vi "Edit_Maths_Equation.vi"(3 "Template Info Array":T1[](array[typedef]) {"Tolerance" min=0.0 format="%#.4f"}, 4 "Maths Equation In":string, 5 "Channel Name":string) -> (0 "Template Info Array Out":T1[](array[typedef]) {"Tolerance" min=0.0 format="%#.4f"}, 1 "Maths Equation Out":string)   [LabVIEW 2013]
uses:
  File_Template_Clus.ctl
panel:
  out "Maths Equation Symbols":string
  in  "Start String":string
  in  "K":u16(ring) items=["Survey:No:", "U(ref)::", "U(ref):Turb:%", "U_{5hp}/U_{ref}::", "Vmag_{5hp}::", "U_{5hp}::", "V_{5hp}::", "W_{5hp}::", "Y_{5hp} (mm)::", "Z_{5hp} (mm)::", "U_{HW}::", "U_{HW}/U_{ref}::", "U_{HW}:Turb:%", "Y_{HW} (mm)::", "Z_{HW} (mm)::", "Date:of:Measurement", "Time:Measurement:Commenced", "Run:Start Time:", "Seconds:since:1st Jan", "Run:Messages:", "Original:Results:Filename", "Raw:Data:Filename", "Reference:Temperature:Used for Corrections", "Atmos:Pressure:Used for Corrections", "Slab Metadata:X-Location:", "Slab Metadata:Floor:", "Slab Metadata:Diverters:", "Slab Metadata:Screens:", "Slab Metadata:TurningVanes:", "Slab Metadata:Deflectors:", "Slab Metadata:MirrorWall:", "Slab Metadata:CloudWall:", "Slab Metadata:DiffuserExit:", "Slab Metadata:ConfigNumber:", "Slab Metadata:ProfileXLocation:", "Slab Metadata:DivererAngle:", "Slab Metadata:DiverterOrientation:", "Slab Metadata:DiverterAngleUpper:", "Slab Metadata:DiverterAngleLower:", "Slab Metadata:DiverterOrientUpper:", "Slab Metadata:DiverterOrientLower:", "Slab Metadata:MirrorWallStandoff:", "Slab Metadata:VertDivWall:", "Slab Metadata:VertDivWindow:", "Ch 0:Variance:Gen (Uref)", "Ch 6:Variance:HW (HW)", "Gen (Uref):Standard Error:in Mean", "Gen (Uref):Standard Error:in Variance", "Ch 1:Mean:Mano (5-1)", "Ch 1:Variance:Mano (5-1)", "Ch 1:SD:Mano (5-1)", "Ch 1:SDonMean:Mano (5-1)", "Ch 2:Mean:Mano (5-2)", "Ch 2:Variance:Mano (5-2)", "Ch 3:Mean:Mano (5-3)", "Ch 3:Variance:Mano (5-3)", "Ch 4:Mean:Mano (5-4)", "Ch 4:Variance:Mano (5-4)", "Ch 5:Mean:Mano (5-5)", "Ch 5:Variance:Mano (5-5)", "HW (HW):Standard Error:in Mean", "HW (HW):Standard Error:in Variance", "HW (HW):Timescale Estimate:Integrated to 25%", "Mode:Plug in:"]
  in  "String 10":string
  in  "J":u16(ring) items=["Survey:No:", "U(ref)::", "U(ref):Turb:%", "U_{5hp}/U_{ref}::", "Vmag_{5hp}::", "U_{5hp}::", "V_{5hp}::", "W_{5hp}::", "Y_{5hp} (mm)::", "Z_{5hp} (mm)::", "U_{HW}::", "U_{HW}/U_{ref}::", "U_{HW}:Turb:%", "Y_{HW} (mm)::", "Z_{HW} (mm)::", "Date:of:Measurement", "Time:Measurement:Commenced", "Run:Start Time:", "Seconds:since:1st Jan", "Run:Messages:", "Original:Results:Filename", "Raw:Data:Filename", "Reference:Temperature:Used for Corrections", "Atmos:Pressure:Used for Corrections", "Slab Metadata:X-Location:", "Slab Metadata:Floor:", "Slab Metadata:Diverters:", "Slab Metadata:Screens:", "Slab Metadata:TurningVanes:", "Slab Metadata:Deflectors:", "Slab Metadata:MirrorWall:", "Slab Metadata:CloudWall:", "Slab Metadata:DiffuserExit:", "Slab Metadata:ConfigNumber:", "Slab Metadata:ProfileXLocation:", "Slab Metadata:DivererAngle:", "Slab Metadata:DiverterOrientation:", "Slab Metadata:DiverterAngleUpper:", "Slab Metadata:DiverterAngleLower:", "Slab Metadata:DiverterOrientUpper:", "Slab Metadata:DiverterOrientLower:", "Slab Metadata:MirrorWallStandoff:", "Slab Metadata:VertDivWall:", "Slab Metadata:VertDivWindow:", "Ch 0:Variance:Gen (Uref)", "Ch 6:Variance:HW (HW)", "Gen (Uref):Standard Error:in Mean", "Gen (Uref):Standard Error:in Variance", "Ch 1:Mean:Mano (5-1)", "Ch 1:Variance:Mano (5-1)", "Ch 1:SD:Mano (5-1)", "Ch 1:SDonMean:Mano (5-1)", "Ch 2:Mean:Mano (5-2)", "Ch 2:Variance:Mano (5-2)", "Ch 3:Mean:Mano (5-3)", "Ch 3:Variance:Mano (5-3)", "Ch 4:Mean:Mano (5-4)", "Ch 4:Variance:Mano (5-4)", "Ch 5:Mean:Mano (5-5)", "Ch 5:Variance:Mano (5-5)", "HW (HW):Standard Error:in Mean", "HW (HW):Standard Error:in Variance", "HW (HW):Timescale Estimate:Integrated to 25%", "Mode:Plug in:"]
  in  "String 9":string
  in  "H":u16(ring) items=["Survey:No:", "U(ref)::", "U(ref):Turb:%", "U_{5hp}/U_{ref}::", "Vmag_{5hp}::", "U_{5hp}::", "V_{5hp}::", "W_{5hp}::", "Y_{5hp} (mm)::", "Z_{5hp} (mm)::", "U_{HW}::", "U_{HW}/U_{ref}::", "U_{HW}:Turb:%", "Y_{HW} (mm)::", "Z_{HW} (mm)::", "Date:of:Measurement", "Time:Measurement:Commenced", "Run:Start Time:", "Seconds:since:1st Jan", "Run:Messages:", "Original:Results:Filename", "Raw:Data:Filename", "Reference:Temperature:Used for Corrections", "Atmos:Pressure:Used for Corrections", "Slab Metadata:X-Location:", "Slab Metadata:Floor:", "Slab Metadata:Diverters:", "Slab Metadata:Screens:", "Slab Metadata:TurningVanes:", "Slab Metadata:Deflectors:", "Slab Metadata:MirrorWall:", "Slab Metadata:CloudWall:", "Slab Metadata:DiffuserExit:", "Slab Metadata:ConfigNumber:", "Slab Metadata:ProfileXLocation:", "Slab Metadata:DivererAngle:", "Slab Metadata:DiverterOrientation:", "Slab Metadata:DiverterAngleUpper:", "Slab Metadata:DiverterAngleLower:", "Slab Metadata:DiverterOrientUpper:", "Slab Metadata:DiverterOrientLower:", "Slab Metadata:MirrorWallStandoff:", "Slab Metadata:VertDivWall:", "Slab Metadata:VertDivWindow:", "Ch 0:Variance:Gen (Uref)", "Ch 6:Variance:HW (HW)", "Gen (Uref):Standard Error:in Mean", "Gen (Uref):Standard Error:in Variance", "Ch 1:Mean:Mano (5-1)", "Ch 1:Variance:Mano (5-1)", "Ch 1:SD:Mano (5-1)", "Ch 1:SDonMean:Mano (5-1)", "Ch 2:Mean:Mano (5-2)", "Ch 2:Variance:Mano (5-2)", "Ch 3:Mean:Mano (5-3)", "Ch 3:Variance:Mano (5-3)", "Ch 4:Mean:Mano (5-4)", "Ch 4:Variance:Mano (5-4)", "Ch 5:Mean:Mano (5-5)", "Ch 5:Variance:Mano (5-5)", "HW (HW):Standard Error:in Mean", "HW (HW):Standard Error:in Variance", "HW (HW):Timescale Estimate:Integrated to 25%", "Mode:Plug in:"]
  in  "String 8":string
  in  "G":u16(ring) items=["Survey:No:", "U(ref)::", "U(ref):Turb:%", "U_{5hp}/U_{ref}::", "Vmag_{5hp}::", "U_{5hp}::", "V_{5hp}::", "W_{5hp}::", "Y_{5hp} (mm)::", "Z_{5hp} (mm)::", "U_{HW}::", "U_{HW}/U_{ref}::", "U_{HW}:Turb:%", "Y_{HW} (mm)::", "Z_{HW} (mm)::", "Date:of:Measurement", "Time:Measurement:Commenced", "Run:Start Time:", "Seconds:since:1st Jan", "Run:Messages:", "Original:Results:Filename", "Raw:Data:Filename", "Reference:Temperature:Used for Corrections", "Atmos:Pressure:Used for Corrections", "Slab Metadata:X-Location:", "Slab Metadata:Floor:", "Slab Metadata:Diverters:", "Slab Metadata:Screens:", "Slab Metadata:TurningVanes:", "Slab Metadata:Deflectors:", "Slab Metadata:MirrorWall:", "Slab Metadata:CloudWall:", "Slab Metadata:DiffuserExit:", "Slab Metadata:ConfigNumber:", "Slab Metadata:ProfileXLocation:", "Slab Metadata:DivererAngle:", "Slab Metadata:DiverterOrientation:", "Slab Metadata:DiverterAngleUpper:", "Slab Metadata:DiverterAngleLower:", "Slab Metadata:DiverterOrientUpper:", "Slab Metadata:DiverterOrientLower:", "Slab Metadata:MirrorWallStandoff:", "Slab Metadata:VertDivWall:", "Slab Metadata:VertDivWindow:", "Ch 0:Variance:Gen (Uref)", "Ch 6:Variance:HW (HW)", "Gen (Uref):Standard Error:in Mean", "Gen (Uref):Standard Error:in Variance", "Ch 1:Mean:Mano (5-1)", "Ch 1:Variance:Mano (5-1)", "Ch 1:SD:Mano (5-1)", "Ch 1:SDonMean:Mano (5-1)", "Ch 2:Mean:Mano (5-2)", "Ch 2:Variance:Mano (5-2)", "Ch 3:Mean:Mano (5-3)", "Ch 3:Variance:Mano (5-3)", "Ch 4:Mean:Mano (5-4)", "Ch 4:Variance:Mano (5-4)", "Ch 5:Mean:Mano (5-5)", "Ch 5:Variance:Mano (5-5)", "HW (HW):Standard Error:in Mean", "HW (HW):Standard Error:in Variance", "HW (HW):Timescale Estimate:Integrated to 25%", "Mode:Plug in:"]
  in  "String 7":string
  in  "F":u16(ring) items=["Survey:No:", "U(ref)::", "U(ref):Turb:%", "U_{5hp}/U_{ref}::", "Vmag_{5hp}::", "U_{5hp}::", "V_{5hp}::", "W_{5hp}::", "Y_{5hp} (mm)::", "Z_{5hp} (mm)::", "U_{HW}::", "U_{HW}/U_{ref}::", "U_{HW}:Turb:%", "Y_{HW} (mm)::", "Z_{HW} (mm)::", "Date:of:Measurement", "Time:Measurement:Commenced", "Run:Start Time:", "Seconds:since:1st Jan", "Run:Messages:", "Original:Results:Filename", "Raw:Data:Filename", "Reference:Temperature:Used for Corrections", "Atmos:Pressure:Used for Corrections", "Slab Metadata:X-Location:", "Slab Metadata:Floor:", "Slab Metadata:Diverters:", "Slab Metadata:Screens:", "Slab Metadata:TurningVanes:", "Slab Metadata:Deflectors:", "Slab Metadata:MirrorWall:", "Slab Metadata:CloudWall:", "Slab Metadata:DiffuserExit:", "Slab Metadata:ConfigNumber:", "Slab Metadata:ProfileXLocation:", "Slab Metadata:DivererAngle:", "Slab Metadata:DiverterOrientation:", "Slab Metadata:DiverterAngleUpper:", "Slab Metadata:DiverterAngleLower:", "Slab Metadata:DiverterOrientUpper:", "Slab Metadata:DiverterOrientLower:", "Slab Metadata:MirrorWallStandoff:", "Slab Metadata:VertDivWall:", "Slab Metadata:VertDivWindow:", "Ch 0:Variance:Gen (Uref)", "Ch 6:Variance:HW (HW)", "Gen (Uref):Standard Error:in Mean", "Gen (Uref):Standard Error:in Variance", "Ch 1:Mean:Mano (5-1)", "Ch 1:Variance:Mano (5-1)", "Ch 1:SD:Mano (5-1)", "Ch 1:SDonMean:Mano (5-1)", "Ch 2:Mean:Mano (5-2)", "Ch 2:Variance:Mano (5-2)", "Ch 3:Mean:Mano (5-3)", "Ch 3:Variance:Mano (5-3)", "Ch 4:Mean:Mano (5-4)", "Ch 4:Variance:Mano (5-4)", "Ch 5:Mean:Mano (5-5)", "Ch 5:Variance:Mano (5-5)", "HW (HW):Standard Error:in Mean", "HW (HW):Standard Error:in Variance", "HW (HW):Timescale Estimate:Integrated to 25%", "Mode:Plug in:"]
  in  "String 6":string
  in  "E":u16(ring) items=["Survey:No:", "U(ref)::", "U(ref):Turb:%", "U_{5hp}/U_{ref}::", "Vmag_{5hp}::", "U_{5hp}::", "V_{5hp}::", "W_{5hp}::", "Y_{5hp} (mm)::", "Z_{5hp} (mm)::", "U_{HW}::", "U_{HW}/U_{ref}::", "U_{HW}:Turb:%", "Y_{HW} (mm)::", "Z_{HW} (mm)::", "Date:of:Measurement", "Time:Measurement:Commenced", "Run:Start Time:", "Seconds:since:1st Jan", "Run:Messages:", "Original:Results:Filename", "Raw:Data:Filename", "Reference:Temperature:Used for Corrections", "Atmos:Pressure:Used for Corrections", "Slab Metadata:X-Location:", "Slab Metadata:Floor:", "Slab Metadata:Diverters:", "Slab Metadata:Screens:", "Slab Metadata:TurningVanes:", "Slab Metadata:Deflectors:", "Slab Metadata:MirrorWall:", "Slab Metadata:CloudWall:", "Slab Metadata:DiffuserExit:", "Slab Metadata:ConfigNumber:", "Slab Metadata:ProfileXLocation:", "Slab Metadata:DivererAngle:", "Slab Metadata:DiverterOrientation:", "Slab Metadata:DiverterAngleUpper:", "Slab Metadata:DiverterAngleLower:", "Slab Metadata:DiverterOrientUpper:", "Slab Metadata:DiverterOrientLower:", "Slab Metadata:MirrorWallStandoff:", "Slab Metadata:VertDivWall:", "Slab Metadata:VertDivWindow:", "Ch 0:Variance:Gen (Uref)", "Ch 6:Variance:HW (HW)", "Gen (Uref):Standard Error:in Mean", "Gen (Uref):Standard Error:in Variance", "Ch 1:Mean:Mano (5-1)", "Ch 1:Variance:Mano (5-1)", "Ch 1:SD:Mano (5-1)", "Ch 1:SDonMean:Mano (5-1)", "Ch 2:Mean:Mano (5-2)", "Ch 2:Variance:Mano (5-2)", "Ch 3:Mean:Mano (5-3)", "Ch 3:Variance:Mano (5-3)", "Ch 4:Mean:Mano (5-4)", "Ch 4:Variance:Mano (5-4)", "Ch 5:Mean:Mano (5-5)", "Ch 5:Variance:Mano (5-5)", "HW (HW):Standard Error:in Mean", "HW (HW):Standard Error:in Variance", "HW (HW):Timescale Estimate:Integrated to 25%", "Mode:Plug in:"]
  in  "String 5":string
  in  "D":u16(ring) items=["Survey:No:", "U(ref)::", "U(ref):Turb:%", "U_{5hp}/U_{ref}::", "Vmag_{5hp}::", "U_{5hp}::", "V_{5hp}::", "W_{5hp}::", "Y_{5hp} (mm)::", "Z_{5hp} (mm)::", "U_{HW}::", "U_{HW}/U_{ref}::", "U_{HW}:Turb:%", "Y_{HW} (mm)::", "Z_{HW} (mm)::", "Date:of:Measurement", "Time:Measurement:Commenced", "Run:Start Time:", "Seconds:since:1st Jan", "Run:Messages:", "Original:Results:Filename", "Raw:Data:Filename", "Reference:Temperature:Used for Corrections", "Atmos:Pressure:Used for Corrections", "Slab Metadata:X-Location:", "Slab Metadata:Floor:", "Slab Metadata:Diverters:", "Slab Metadata:Screens:", "Slab Metadata:TurningVanes:", "Slab Metadata:Deflectors:", "Slab Metadata:MirrorWall:", "Slab Metadata:CloudWall:", "Slab Metadata:DiffuserExit:", "Slab Metadata:ConfigNumber:", "Slab Metadata:ProfileXLocation:", "Slab Metadata:DivererAngle:", "Slab Metadata:DiverterOrientation:", "Slab Metadata:DiverterAngleUpper:", "Slab Metadata:DiverterAngleLower:", "Slab Metadata:DiverterOrientUpper:", "Slab Metadata:DiverterOrientLower:", "Slab Metadata:MirrorWallStandoff:", "Slab Metadata:VertDivWall:", "Slab Metadata:VertDivWindow:", "Ch 0:Variance:Gen (Uref)", "Ch 6:Variance:HW (HW)", "Gen (Uref):Standard Error:in Mean", "Gen (Uref):Standard Error:in Variance", "Ch 1:Mean:Mano (5-1)", "Ch 1:Variance:Mano (5-1)", "Ch 1:SD:Mano (5-1)", "Ch 1:SDonMean:Mano (5-1)", "Ch 2:Mean:Mano (5-2)", "Ch 2:Variance:Mano (5-2)", "Ch 3:Mean:Mano (5-3)", "Ch 3:Variance:Mano (5-3)", "Ch 4:Mean:Mano (5-4)", "Ch 4:Variance:Mano (5-4)", "Ch 5:Mean:Mano (5-5)", "Ch 5:Variance:Mano (5-5)", "HW (HW):Standard Error:in Mean", "HW (HW):Standard Error:in Variance", "HW (HW):Timescale Estimate:Integrated to 25%", "Mode:Plug in:"]
  in  "String 4":string
  in  "C":u16(ring) items=["Survey:No:", "U(ref)::", "U(ref):Turb:%", "U_{5hp}/U_{ref}::", "Vmag_{5hp}::", "U_{5hp}::", "V_{5hp}::", "W_{5hp}::", "Y_{5hp} (mm)::", "Z_{5hp} (mm)::", "U_{HW}::", "U_{HW}/U_{ref}::", "U_{HW}:Turb:%", "Y_{HW} (mm)::", "Z_{HW} (mm)::", "Date:of:Measurement", "Time:Measurement:Commenced", "Run:Start Time:", "Seconds:since:1st Jan", "Run:Messages:", "Original:Results:Filename", "Raw:Data:Filename", "Reference:Temperature:Used for Corrections", "Atmos:Pressure:Used for Corrections", "Slab Metadata:X-Location:", "Slab Metadata:Floor:", "Slab Metadata:Diverters:", "Slab Metadata:Screens:", "Slab Metadata:TurningVanes:", "Slab Metadata:Deflectors:", "Slab Metadata:MirrorWall:", "Slab Metadata:CloudWall:", "Slab Metadata:DiffuserExit:", "Slab Metadata:ConfigNumber:", "Slab Metadata:ProfileXLocation:", "Slab Metadata:DivererAngle:", "Slab Metadata:DiverterOrientation:", "Slab Metadata:DiverterAngleUpper:", "Slab Metadata:DiverterAngleLower:", "Slab Metadata:DiverterOrientUpper:", "Slab Metadata:DiverterOrientLower:", "Slab Metadata:MirrorWallStandoff:", "Slab Metadata:VertDivWall:", "Slab Metadata:VertDivWindow:", "Ch 0:Variance:Gen (Uref)", "Ch 6:Variance:HW (HW)", "Gen (Uref):Standard Error:in Mean", "Gen (Uref):Standard Error:in Variance", "Ch 1:Mean:Mano (5-1)", "Ch 1:Variance:Mano (5-1)", "Ch 1:SD:Mano (5-1)", "Ch 1:SDonMean:Mano (5-1)", "Ch 2:Mean:Mano (5-2)", "Ch 2:Variance:Mano (5-2)", "Ch 3:Mean:Mano (5-3)", "Ch 3:Variance:Mano (5-3)", "Ch 4:Mean:Mano (5-4)", "Ch 4:Variance:Mano (5-4)", "Ch 5:Mean:Mano (5-5)", "Ch 5:Variance:Mano (5-5)", "HW (HW):Standard Error:in Mean", "HW (HW):Standard Error:in Variance", "HW (HW):Timescale Estimate:Integrated to 25%", "Mode:Plug in:"]
  in  "String 3":string
  in  "B":u16(ring) items=["Survey:No:", "U(ref)::", "U(ref):Turb:%", "U_{5hp}/U_{ref}::", "Vmag_{5hp}::", "U_{5hp}::", "V_{5hp}::", "W_{5hp}::", "Y_{5hp} (mm)::", "Z_{5hp} (mm)::", "U_{HW}::", "U_{HW}/U_{ref}::", "U_{HW}:Turb:%", "Y_{HW} (mm)::", "Z_{HW} (mm)::", "Date:of:Measurement", "Time:Measurement:Commenced", "Run:Start Time:", "Seconds:since:1st Jan", "Run:Messages:", "Original:Results:Filename", "Raw:Data:Filename", "Reference:Temperature:Used for Corrections", "Atmos:Pressure:Used for Corrections", "Slab Metadata:X-Location:", "Slab Metadata:Floor:", "Slab Metadata:Diverters:", "Slab Metadata:Screens:", "Slab Metadata:TurningVanes:", "Slab Metadata:Deflectors:", "Slab Metadata:MirrorWall:", "Slab Metadata:CloudWall:", "Slab Metadata:DiffuserExit:", "Slab Metadata:ConfigNumber:", "Slab Metadata:ProfileXLocation:", "Slab Metadata:DivererAngle:", "Slab Metadata:DiverterOrientation:", "Slab Metadata:DiverterAngleUpper:", "Slab Metadata:DiverterAngleLower:", "Slab Metadata:DiverterOrientUpper:", "Slab Metadata:DiverterOrientLower:", "Slab Metadata:MirrorWallStandoff:", "Slab Metadata:VertDivWall:", "Slab Metadata:VertDivWindow:", "Ch 0:Variance:Gen (Uref)", "Ch 6:Variance:HW (HW)", "Gen (Uref):Standard Error:in Mean", "Gen (Uref):Standard Error:in Variance", "Ch 1:Mean:Mano (5-1)", "Ch 1:Variance:Mano (5-1)", "Ch 1:SD:Mano (5-1)", "Ch 1:SDonMean:Mano (5-1)", "Ch 2:Mean:Mano (5-2)", "Ch 2:Variance:Mano (5-2)", "Ch 3:Mean:Mano (5-3)", "Ch 3:Variance:Mano (5-3)", "Ch 4:Mean:Mano (5-4)", "Ch 4:Variance:Mano (5-4)", "Ch 5:Mean:Mano (5-5)", "Ch 5:Variance:Mano (5-5)", "HW (HW):Standard Error:in Mean", "HW (HW):Standard Error:in Variance", "HW (HW):Timescale Estimate:Integrated to 25%", "Mode:Plug in:"]
  in  "String 2":string
  in  "A":u16(ring) items=["Survey:No:", "U(ref)::", "U(ref):Turb:%", "U_{5hp}/U_{ref}::", "Vmag_{5hp}::", "U_{5hp}::", "V_{5hp}::", "W_{5hp}::", "Y_{5hp} (mm)::", "Z_{5hp} (mm)::", "U_{HW}::", "U_{HW}/U_{ref}::", "U_{HW}:Turb:%", "Y_{HW} (mm)::", "Z_{HW} (mm)::", "Date:of:Measurement", "Time:Measurement:Commenced", "Run:Start Time:", "Seconds:since:1st Jan", "Run:Messages:", "Original:Results:Filename", "Raw:Data:Filename", "Reference:Temperature:Used for Corrections", "Atmos:Pressure:Used for Corrections", "Slab Metadata:X-Location:", "Slab Metadata:Floor:", "Slab Metadata:Diverters:", "Slab Metadata:Screens:", "Slab Metadata:TurningVanes:", "Slab Metadata:Deflectors:", "Slab Metadata:MirrorWall:", "Slab Metadata:CloudWall:", "Slab Metadata:DiffuserExit:", "Slab Metadata:ConfigNumber:", "Slab Metadata:ProfileXLocation:", "Slab Metadata:DivererAngle:", "Slab Metadata:DiverterOrientation:", "Slab Metadata:DiverterAngleUpper:", "Slab Metadata:DiverterAngleLower:", "Slab Metadata:DiverterOrientUpper:", "Slab Metadata:DiverterOrientLower:", "Slab Metadata:MirrorWallStandoff:", "Slab Metadata:VertDivWall:", "Slab Metadata:VertDivWindow:", "Ch 0:Variance:Gen (Uref)", "Ch 6:Variance:HW (HW)", "Gen (Uref):Standard Error:in Mean", "Gen (Uref):Standard Error:in Variance", "Ch 1:Mean:Mano (5-1)", "Ch 1:Variance:Mano (5-1)", "Ch 1:SD:Mano (5-1)", "Ch 1:SDonMean:Mano (5-1)", "Ch 2:Mean:Mano (5-2)", "Ch 2:Variance:Mano (5-2)", "Ch 3:Mean:Mano (5-3)", "Ch 3:Variance:Mano (5-3)", "Ch 4:Mean:Mano (5-4)", "Ch 4:Variance:Mano (5-4)", "Ch 5:Mean:Mano (5-5)", "Ch 5:Variance:Mano (5-5)", "HW (HW):Standard Error:in Mean", "HW (HW):Standard Error:in Variance", "HW (HW):Timescale Estimate:Integrated to 25%", "Mode:Plug in:"]
  in  "String 1":string
  in  "Reset":bool
  in  "Number of Variables":i32
  in  "OK":bool
  # "> 20  or\n<20   or\n =20"
  # "<<Characters_to_Match>>  <<Replace_Whole_String_with_this>>"
  # "<<Channel_Name>> contains <<Characters to match>> or\n<<Channel_Name>> does not contain <<Characters to match>>"
  # "<<Channel_Name_A>> + <<Channel_Name_B>> or\nConcatenate <<Channel_Name_A>> and <<Channel_Name_B>>"
  # "> 20  or\n<20   or\n =20"
  # "<<Characters_to_Match>>  <<Replace_Whole_String_with_this>>"
  # "<<Channel_Name>> contains <<Characters to match>> or\n<<Channel_Name>> does not contain <<Characters to match>>"
  # "<<Channel_Name_A>> + <<Channel_Name_B>> or\nConcatenate <<Channel_Name_A>> and <<Channel_Name_B>>"
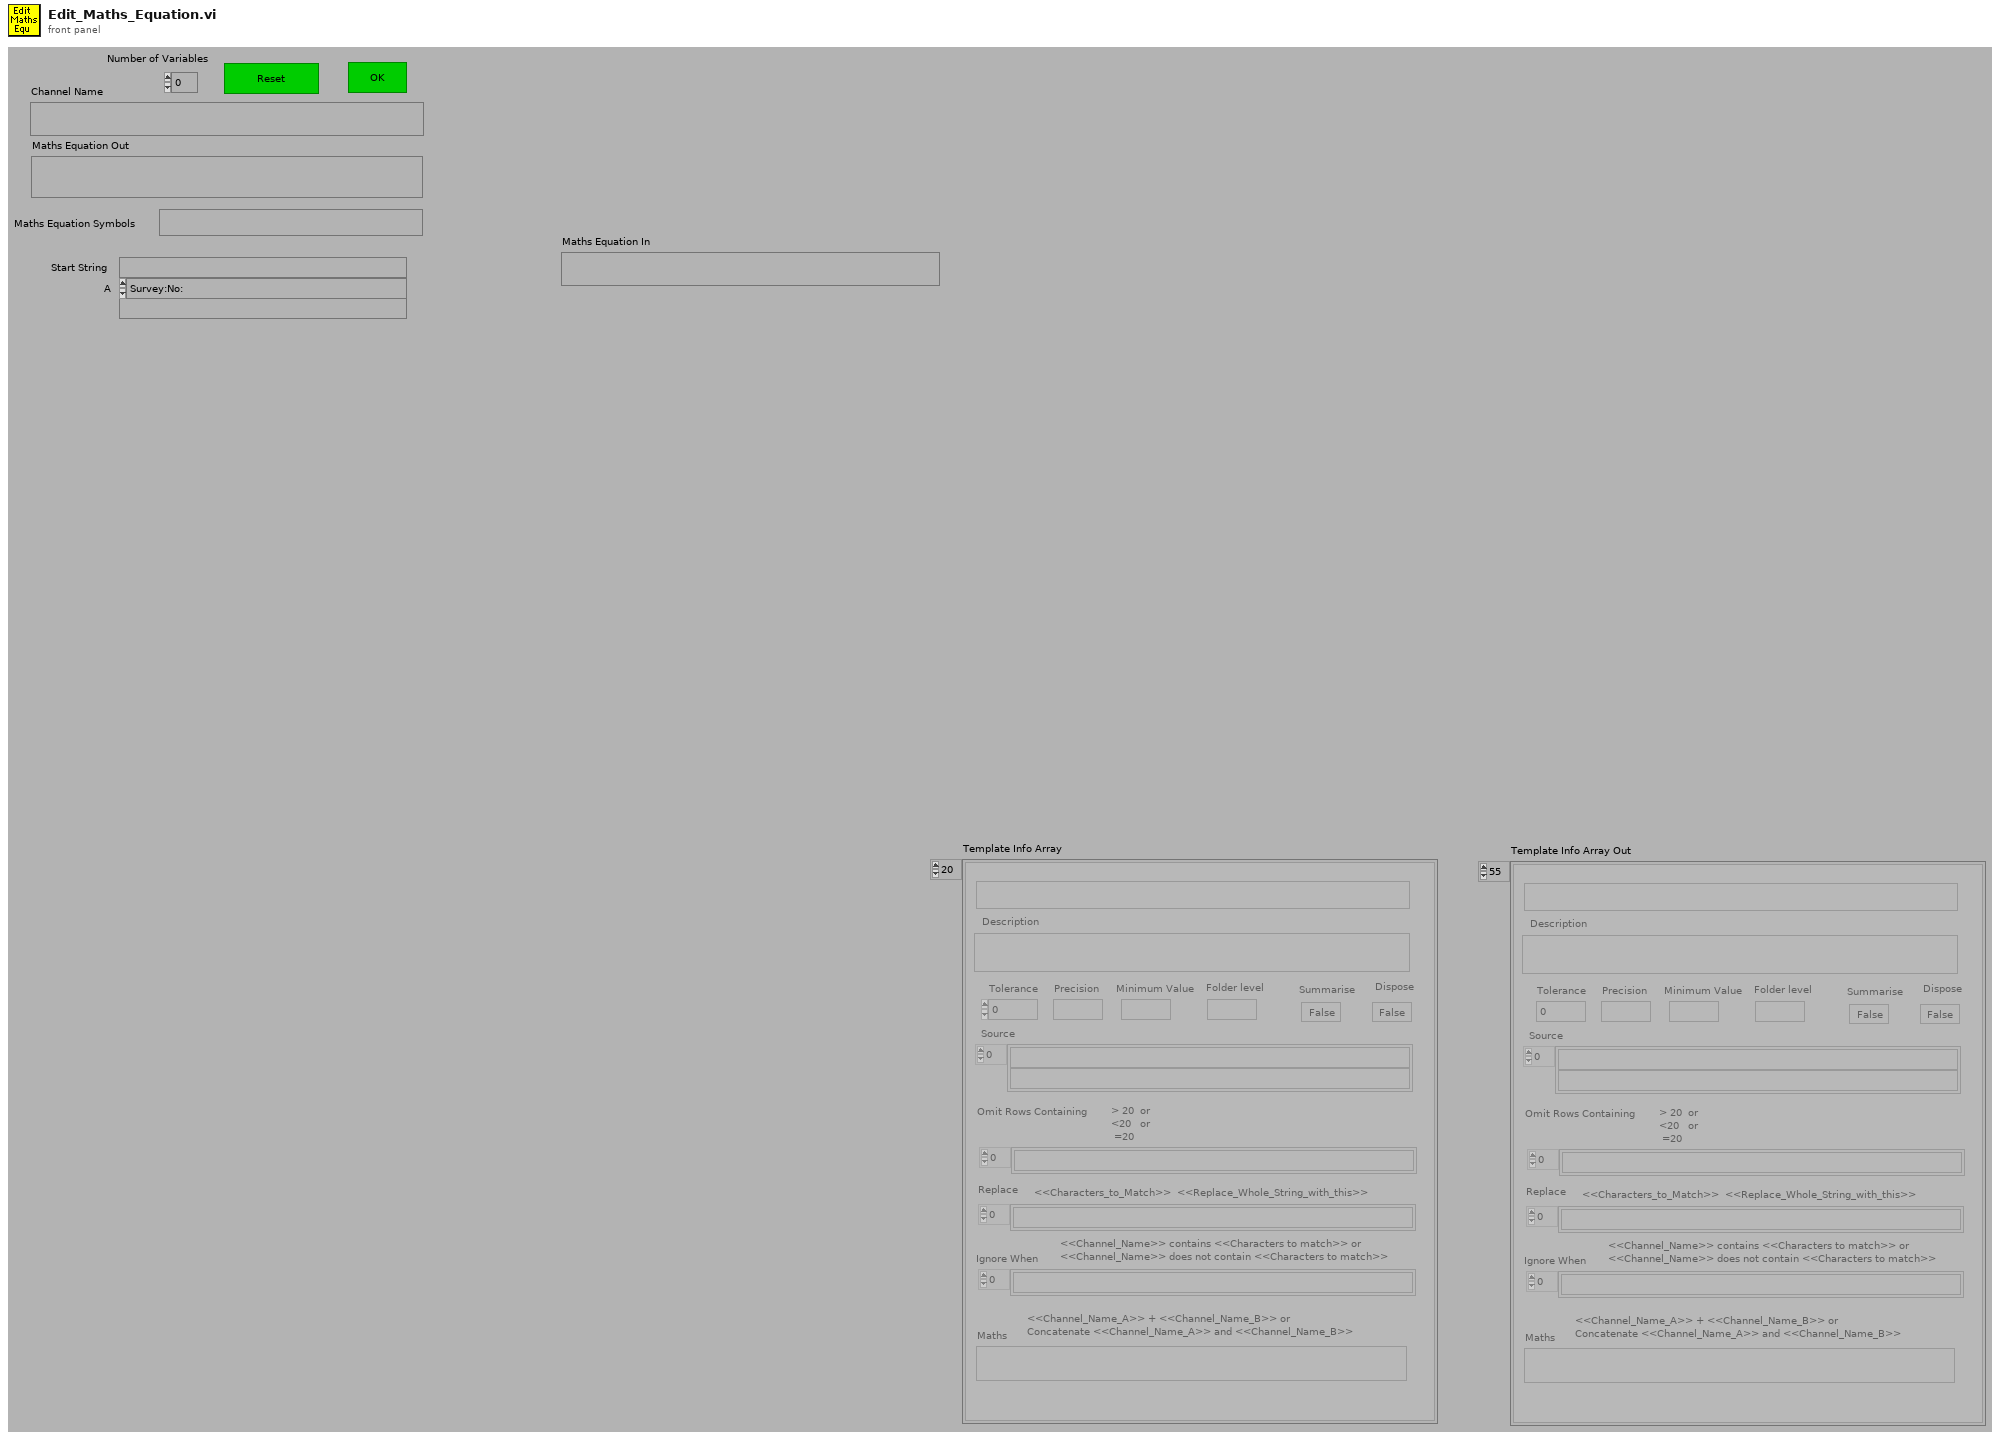
[diagram p1: front panel]
types:
  T1 = typedef "File_Template_Clus.ctl" = cluster{"Template Channel Name":string, "Description":string, "Tolerance":dbl, "Precision":string, "Folder level":string, "Source":string[], "Replace":string[], "Summarise":bool, "Dispose":bool, "Minimum Value":string, "Maths":string, "Omit Rows Containing":string[], "Ignore When":string[]}
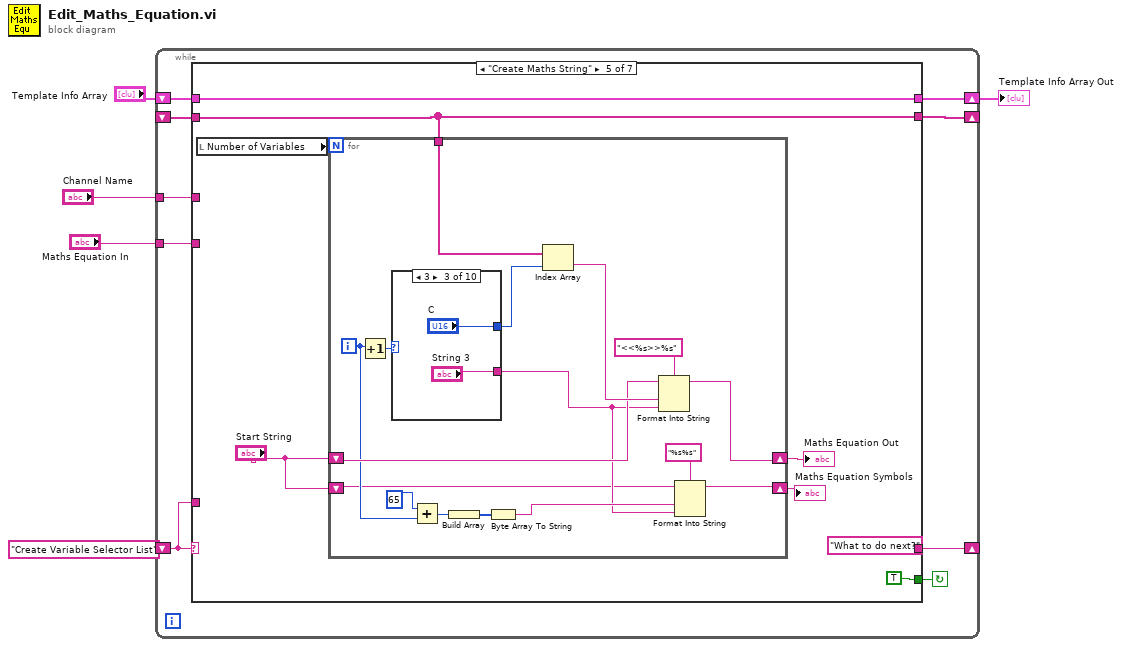
[diagram p0: block diagram]
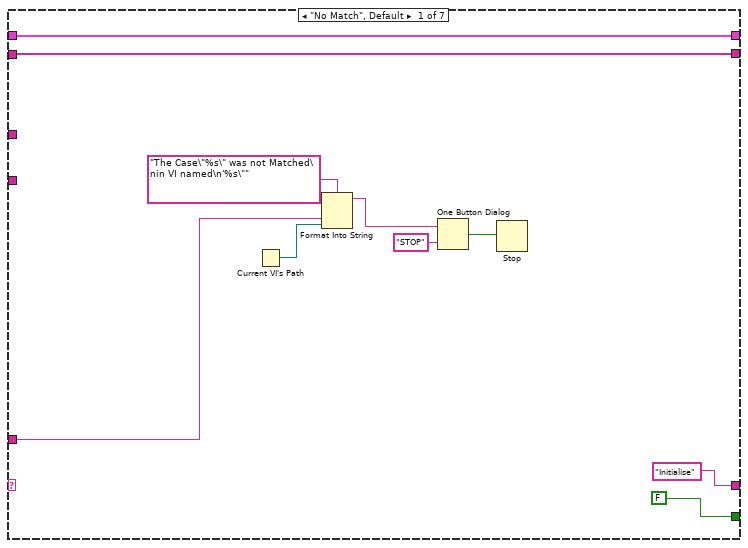
[diagram p2: hidden frame]
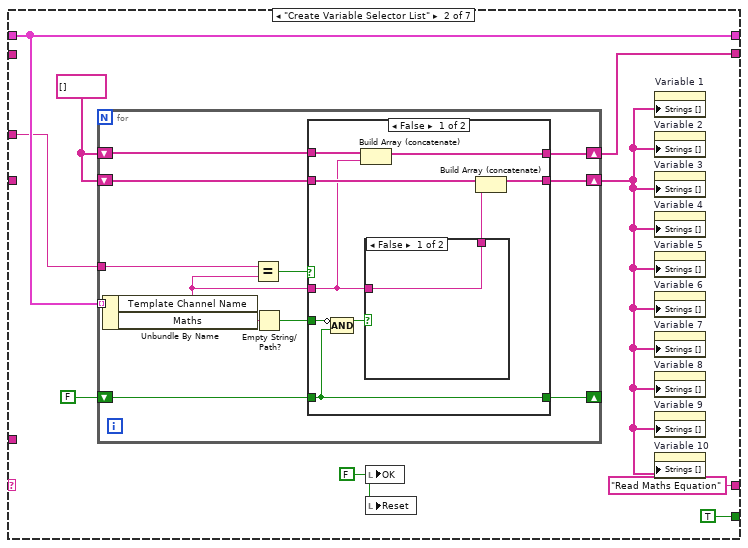
[diagram p3: hidden frame]
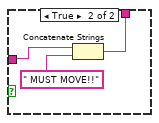
[diagram p4: hidden frame]
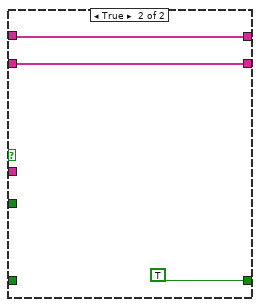
[diagram p5: hidden frame]
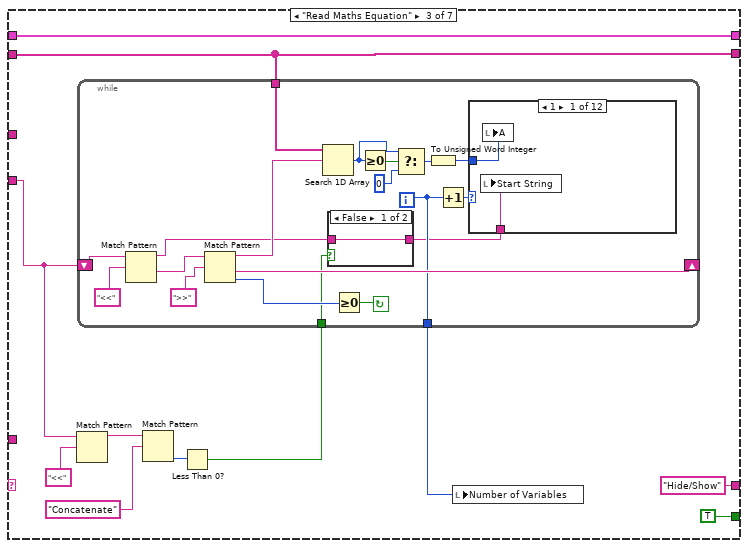
[diagram p6: hidden frame]
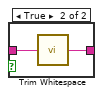
[diagram p7: hidden frame]
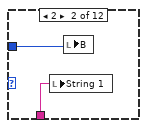
[diagram p8: hidden frame]
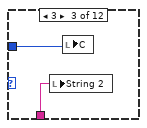
[diagram p9: hidden frame]
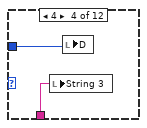
[diagram p10: hidden frame]
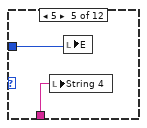
[diagram p11: hidden frame]
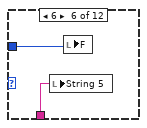
[diagram p12: hidden frame]
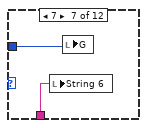
[diagram p13: hidden frame]
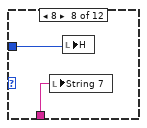
[diagram p14: hidden frame]
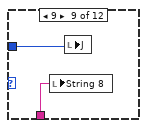
[diagram p15: hidden frame]
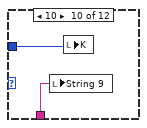
[diagram p16: hidden frame]
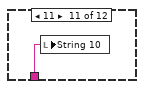
[diagram p17: hidden frame]
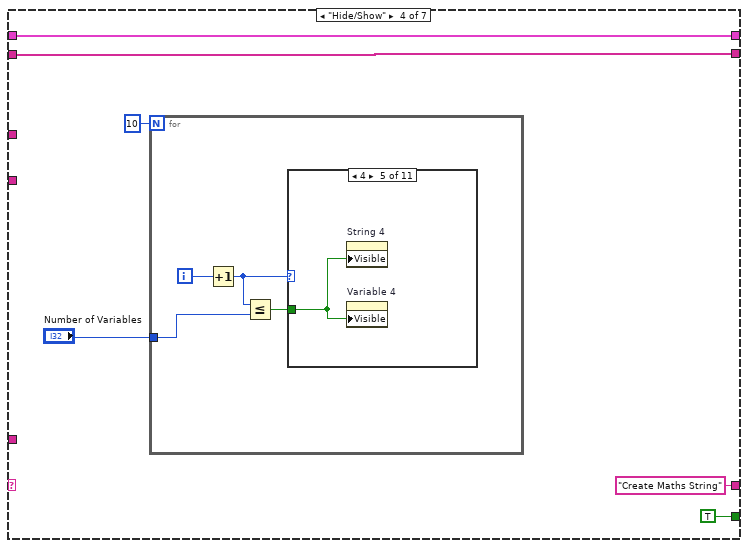
[diagram p19: hidden frame]
diagram:
  n1 = while {
    tunnel: "Channel Name" -> [w6]
    tunnel: "Maths Equation In" -> [w7]
    shift-left: _ -> [w8]
    shift-right: [w9] -> _
    shift-left: "Template Info Array" -> [w10]
    shift-right: [w11] -> w3
    shift-left: "Create Variable Selector List" -> [w12]
    shift-right: [w13] -> _
    stop <- w14 continue-if-true
    n2 = case shown="\"Create Maths String\"" w12 {
      tunnel: [FALSE TRUE TRUE TRUE TRUE TRUE FALSE] -> w14
      tunnel: ["Initialise" "Read Maths Equation" "Hide/Show" "Create Maths String" "What to do next?" w181 "End"] -> w13
      tunnel: w12 -> [w19 _ _ _ _ _ _]
      tunnel: [w16 w32 w71 w120 w141 w191 w200] -> w11
      tunnel: w10 -> [w16 w32 w71 w120 w141 w191 w200]
      tunnel: [w15 w30 w70 w119 w139 w185 w199] -> w9
      tunnel: w8 -> [w15 _ w70 w119 w139 w185 w199]
      tunnel: w7 -> [_ _ w66 _ _ _ _]
      tunnel: w6 -> [_ w31 _ _ _ _ _]
      frame "No Match", Default {
        n3 = Current VI's Path() -> (path=w18:path)
        n4 = Format Into String(format string="The Case\"%s\" was not Matched\nin VI named\n'%s\"" ("Format String"), w19, w18) -> (resulting string=w22:string)  [unwired: 2 in, 1 out]
        n5 = One Button Dialog(message=w22, button name ("OK")="STOP") -> (true=w20:bool)
        n6 = Stop(stop? (T)=w20) -> ()
      }
      frame "Create Variable Selector List" {
        w25 = FALSE ("OK")
        w28 = string[] []
        n7 = for {
          shift-right: [w40] -> w30
          shift-left: w28 -> [w42]
          shift-right: [w36] -> w27
          shift-left: w28 -> [w37]
          tunnel: w32 -> [w45] mode=indexing
          tunnel: w31 -> [w44]
          shift-right: [w35] -> _
          shift-left: FALSE -> [w34]
          n8 = Unbundle By Name(w45) -> ("Template Channel Name"=w41:string, "Maths"=w39:string)
          n9 = Equal?(x=w44, y=w41) -> (x = y?=w43:bool)
          n10 = Empty String/Path?(string/path=w39) -> (empty?=w38:bool)
          n11 = case shown="False" w43 {
            tunnel: w42 -> [w54 w60]
            tunnel: w41 -> [w49 _]
            tunnel: [w53 w60] -> w40
            tunnel: w38 -> [w48 _]
            tunnel: w37 -> [w52 w59]
            tunnel: [w51 w59] -> w36
            tunnel: [w46 TRUE] -> w35
            tunnel: w34 -> [w46 _]
            frame False {
              n12 = Compound Arithmetic op=AND(invert w48, w46) -> (w47:bool)
              n13 = Build Array (concatenate)(w54, w49) -> (w53:string[])
              n14 = case shown="False" w47 {
                tunnel: [w55 w57] -> w50
                tunnel: w49 -> [w55 w58]
                frame False {
                }
                frame True {
                  n15 = Concatenate Strings(w58, " MUST MOVE!!" ("Substring")) -> (w57:string)
                }
              }
              n16 = Build Array (concatenate)(w52, w50) -> (w51:string[])
            }
            frame True {
            }
          }
        }
        n17 = local write "OK"(w25) -> ()
        n18 = local write "Reset"(w25) -> ()
        n19 = property on="Variable 1" class="Ring (strict)"("Strings []"=w27) -> ()  [unwired: 2 in, 2 out]
        n20 = property on="Variable 2" class="Ring (strict)"("Strings []"=w27) -> ()  [unwired: 2 in, 2 out]
        n21 = property on="Variable 3" class="Ring (strict)"("Strings []"=w27) -> ()  [unwired: 2 in, 2 out]
        n22 = property on="Variable 4" class="Ring (strict)"("Strings []"=w27) -> ()  [unwired: 2 in, 2 out]
        n23 = property on="Variable 5" class="Ring (strict)"("Strings []"=w27) -> ()  [unwired: 2 in, 2 out]
        n24 = property on="Variable 6" class="Ring (strict)"("Strings []"=w27) -> ()  [unwired: 2 in, 2 out]
        n25 = property on="Variable 7" class="Ring (strict)"("Strings []"=w27) -> ()  [unwired: 2 in, 2 out]
        n26 = property on="Variable 8" class="Ring (strict)"("Strings []"=w27) -> ()  [unwired: 2 in, 2 out]
        n27 = property on="Variable 9" class="Ring (strict)"("Strings []"=w27) -> ()  [unwired: 2 in, 2 out]
        n28 = property on="Variable 10" class="Ring (strict)"("Strings []"=w27) -> ()  [unwired: 2 in, 2 out]
      }
      frame "Read Maths Equation" {
        n29 = Match Pattern(string=w66, regular expression="<<") -> (before substring=w65:string)  [unwired: 4 out]
        n30 = Match Pattern(string=w65, regular expression="Concatenate") -> (offset past match=w63:i32)  [unwired: 4 out]
        n31 = Less Than 0?(x=w63) -> (x < 0?=w62:bool)
        n32 = while {
          tunnel: [w79] -> w69
          tunnel: w70 -> [w88]
          shift-left: w66 -> [w91]
          shift-right: [w81] -> _
          tunnel: w62 -> [w73]
          i -> [w79]
          stop <- w89 continue-if-true
          n33 = Match Pattern(string=w91, regular expression="<<") -> (before substring=w77:string, after substring=w90:string)  [unwired: 3 out]
          n34 = Match Pattern(string=w90, regular expression=">>") -> (before substring=w87:string, after substring=w81:string, offset past match=w80:i32)  [unwired: 2 out]
          n35 = Search 1D Array(1D array=w88, element=w87) -> (index of element=w85:i32)  [unwired: 1 out]
          n36 = case shown="False" w73 {
            tunnel: w77 -> [w92 w94]
            tunnel: [w92 w93] -> w76
            frame False {
            }
            frame True {
              n37 = call <vilib>:"Trim Whitespace.vi"("string"=w94) -> ("trimmed string"=w93:string)  [unwired: 1 in]
            }
          }
          n38 = Greater Or Equal To 0?(x=w80) -> (x >= 0?=w89:bool)
          n39 = Greater Or Equal To 0?(x=w85) -> (x >= 0?=w86:bool)
          n40 = Select(t=w85, s=w86, f=0) -> (s? t:f=w82:i32)
          n41 = To Unsigned Word Integer(number=w82) -> (unsigned 16bit integer=w78:u16)
          n42 = Increment(x=w79) -> (x+1=w83:i32)
          n43 = case shown="1" w83 {
            tunnel: w78 -> [w96 w98 w100 w102 w104 w106 w108 w110 w112 w114 _ _]
            tunnel: w76 -> [w95 w97 w99 w101 w103 w105 w107 w109 w111 w113 w115 _]
            frame 1 {
              n44 = local write "Start String"(w95) -> ()
              n45 = local write "A"(w96) -> ()
            }
            frame 2 {
              n46 = local write "String 1"(w97) -> ()
              n47 = local write "B"(w98) -> ()
            }
            frame 3 {
              n48 = local write "String 2"(w99) -> ()
              n49 = local write "C"(w100) -> ()
            }
            frame 4 {
              n50 = local write "String 3"(w101) -> ()
              n51 = local write "D"(w102) -> ()
            }
            frame 5 {
              n52 = local write "String 4"(w103) -> ()
              n53 = local write "E"(w104) -> ()
            }
            frame 6 {
              n54 = local write "String 5"(w105) -> ()
              n55 = local write "F"(w106) -> ()
            }
            frame 7 {
              n56 = local write "String 6"(w107) -> ()
              n57 = local write "G"(w108) -> ()
            }
            frame 8 {
              n58 = local write "String 7"(w109) -> ()
              n59 = local write "H"(w110) -> ()
            }
            frame 9 {
              n60 = local write "String 8"(w111) -> ()
              n61 = local write "J"(w112) -> ()
            }
            frame 10 {
              n62 = local write "String 9"(w113) -> ()
              n63 = local write "K"(w114) -> ()
            }
            frame 11 {
              n64 = local write "String 10"(w115) -> ()
            }
            frame 12, Default {
            }
          }
        }
        n65 = local write "Number of Variables"(w69) -> ()
      }
      frame "Hide/Show" {
        n66 = for {
          N: 10 -> [_]
          tunnel: "Number of Variables" -> [w123]
          i -> [w125]
          n67 = Increment(x=w125) -> (x+1=w124:i32)
          n68 = Less Or Equal?(x=w124, y=w123) -> (x <= y?=w122:bool)
          n69 = case shown="4" w124 {
            tunnel: w122 -> [_ w126 w127 w128 w129 w130 w131 w132 w133 w134 w135]
            frame 0, Default {
            }
            frame 1 {
              n70 = property on="Variable 1" class="Ring (strict)"("Visible"=w126) -> ()  [unwired: 2 in, 2 out]
              n71 = property on="String 1" class="Str"("Visible"=w126) -> ()  [unwired: 2 in, 2 out]
            }
            frame 2 {
              n72 = property on="Variable 2" class="Ring (strict)"("Visible"=w127) -> ()  [unwired: 2 in, 2 out]
              n73 = property on="String 2" class="Str"("Visible"=w127) -> ()  [unwired: 2 in, 2 out]
            }
            frame 3 {
              n74 = property on="Variable 3" class="Ring (strict)"("Visible"=w128) -> ()  [unwired: 2 in, 2 out]
              n75 = property on="String 3" class="Str"("Visible"=w128) -> ()  [unwired: 2 in, 2 out]
            }
            frame 4 {
              n76 = property on="String 4" class="Str"("Visible"=w129) -> ()  [unwired: 2 in, 2 out]
              n77 = property on="Variable 4" class="Ring (strict)"("Visible"=w129) -> ()  [unwired: 2 in, 2 out]
            }
            frame 5 {
              n78 = property on="String 5" class="Str"("Visible"=w130) -> ()  [unwired: 2 in, 2 out]
              n79 = property on="Variable 5" class="Ring (strict)"("Visible"=w130) -> ()  [unwired: 2 in, 2 out]
            }
            frame 6 {
              n80 = property on="String 6" class="Str"("Visible"=w131) -> ()  [unwired: 2 in, 2 out]
              n81 = property on="Variable 6" class="Ring (strict)"("Visible"=w131) -> ()  [unwired: 2 in, 2 out]
            }
            frame 7 {
              n82 = property on="Variable 7" class="Ring (strict)"("Visible"=w132) -> ()  [unwired: 2 in, 2 out]
              n83 = property on="String 7" class="Str"("Visible"=w132) -> ()  [unwired: 2 in, 2 out]
            }
            frame 8 {
              n84 = property on="String 8" class="Str"("Visible"=w133) -> ()  [unwired: 2 in, 2 out]
              n85 = property on="Variable 8" class="Ring (strict)"("Visible"=w133) -> ()  [unwired: 2 in, 2 out]
            }
            frame 9 {
              n86 = property on="String 9" class="Str"("Visible"=w134) -> ()  [unwired: 2 in, 2 out]
              n87 = property on="Variable 9" class="Ring (strict)"("Visible"=w134) -> ()  [unwired: 2 in, 2 out]
            }
            frame 10 {
              n88 = property on="Variable 10" class="Ring (strict)"("Visible"=w135) -> ()  [unwired: 2 in, 2 out]
              n89 = property on="String 10" class="Str"("Visible"=w135) -> ()  [unwired: 2 in, 2 out]
            }
          }
        }
      }
      frame "Create Maths String" {
        n90 = local read "Number of Variables"() -> (w140:i32)
        n91 = for {
          N: w140 -> [_]
          shift-right: [w154] -> w138
          shift-left: "Start String" -> [w155]
          tunnel: w139 -> [w159]
          shift-right: [w144] -> w136
          shift-left: "Start String" -> [w145]
          i -> [w149]
          n92 = Increment(x=w149) -> (x+1=w157:i32)
          n93 = case shown="3" w157 {
            tunnel: ["A" "B" "C" "D" "E" "F" "G" "H" "J" "K"] -> w158
            tunnel: ["String 1" "String 2" "String 3" "String 4" "String 5" "String 6" "String 7" "String 8" "String 9" "String 10"] -> w146
            frame 1, Default {
            }
            frame 2 {
            }
            frame 3 {
            }
            frame 4 {
            }
            frame 5 {
            }
            frame 6 {
            }
            frame 7 {
            }
            frame 8 {
            }
            frame 9 {
            }
            frame 10 {
            }
          }
          n94 = Add(x=65, y=w149) -> (x+y=w151:i32)
          n95 = Build Array(w151) -> (w152:i32[])
          n96 = Byte Array To String(unsigned byte array=w152) -> (string=w147:string)
          n97 = Index Array(array=w159, index=w158) -> (element=w156:string)
          n98 = Format Into String(format string="<<%s>>%s" ("Format String"), initial string=w155, w156, w146) -> (resulting string=w154:string)  [unwired: 1 in, 1 out]
          n99 = Format Into String(format string="%s%s" ("Format String"), initial string=w145, w147, w146) -> (resulting string=w144:string)  [unwired: 1 in, 1 out]
        }
        "Maths Equation Out" <- w138
        "Maths Equation Symbols" <- w136
      }
      frame "What to do next?" {
        n100 = while {
          tunnel: [w196] -> w189
          shift-left: _ -> [w196]
          shift-right: [w197] -> w190
          stop <- FALSE continue-if-true
          n101 = local read "Number of Variables"() -> (w197:i32)
        }
        n102 = Not Equal?(x=w190, y=w189) -> (x != y?=w186:bool)
        n103 = Select(t="Hide/Show", s=w186, f="Create Maths String") -> (s? t:f=w180:string)
        n104 = Select(t="End", s="OK", f=w180) -> (s? t:f=w182:string)
        n105 = Select(t="Read Maths Equation", s="Reset", f=w182) -> (s? t:f=w181:string)
      }
      frame "End" {
      }
    }
  }
  "Template Info Array Out" <- w3
